vi "TestMain.vi"() -> ()   [LabVIEW 2019]
uses:
  <vilib>/Platform/TimedLoop/XDataNode/timing_clust.ctl
  <vilib>/Platform/TimedLoop/XDataNode/nitl_modes.ctl
  <vilib>/Platform/TimedLoop/XDataNode/wakeup.ctl
  <vilib>/myRIO/Instrument Drivers/Onboard IO/PWM/typedefs/PWM Reference.ctl
  <vilib>/myRIO/Common/Instrument Driver Framework/Utilities/typedefs/myRIO Generic Hardware Reference.ctl
  <vilib>/myRIO/Common/Instrument Driver Framework/Utilities/typedefs/Hardware Version Enum.ctl
  <vilib>/myRIO/Common/Instrument Driver Framework/Utilities/typedefs/myRIO v1.0 Reference.ctl
  <vilib>/myRIO/Common/Instrument Driver Framework/Utilities/typedefs/Generic FPGA Reference.ctl
  <vilib>/myRIO/Common/Instrument Driver Framework/myRIO v1.0/PWM/typedefs/PWM Channels Enum.ctl
  <vilib>/myRIO/Instrument Drivers/Onboard IO/PWM/typedefs/PWM Configuration.ctl
  <vilib>/userDefined/High Color/nirio_resource_hc.ctl
  <vilib>/myRIO/Instrument Drivers/Onboard IO/DIO/typedefs/DIO Reference.ctl
  <vilib>/myRIO/Common/Instrument Driver Framework/myRIO v1.0/DIO/typedefs/DIO Channels List.ctl
  <vilib>/myRIO/Common/Instrument Driver Framework/myRIO v1.0/DIO/typedefs/DIO Channels Enum.ctl
  <vilib>/myRIO/Common/Instrument Driver Framework/Utilities/vis/Is FPGA Ref Available.vi
  <vilib>/myRIO/Common/Instrument Driver Framework/myRIO v1.0/PWM/vis/myRIO v1.1 Open PWM.vi
  <vilib>/myRIO/Instrument Drivers/Onboard IO/PWM/vis/Set Duty Cycle and Frequency.vi
  <vilib>/myRIO/Common/Instrument Driver Framework/myRIO v1.0/DIO/vis/myRIO v1.1 Open DIO.vi
  <extravilib>/ChannelInstances/Tag-bool/Write With Abort.vi
  <extravilib>/ChannelInstances/Tag-bool/Read With Abort.vi
  <vilib>/myRIO/Common/Instrument Driver Framework/Utilities/vis/Validate Channels.vi
  <vilib>/myRIO/Common/Instrument Driver Framework/myRIO v1.0/PWM/vis/myRIO v1.0 Reserve PWM.vi
  <vilib>/myRIO/Common/Instrument Driver Framework/myRIO v1.0/DIO/vis/myRIO v1.0 Reserve DIO.vi
  <vilib>/myRIO/Common/Instrument Driver Framework/myRIO v1.0/I2C/vis/myRIO v1.0 Close I2C.vi
  <vilib>/myRIO/Common/Instrument Driver Framework/myRIO v1.0/UART/vis/myRIO v1.0 Close UART.vi
  <vilib>/myRIO/Common/Instrument Driver Framework/myRIO v1.0/PWM/vis/myRIO v1.0 Build MUX Configuration PWM.vi
  <vilib>/myRIO/Common/Instrument Driver Framework/myRIO v1.0/Resource Manager/vis/myRIO v1.0 Reserve Channel List.vi
  <vilib>/myRIO/Common/Instrument Driver Framework/myRIO v1.0/DIO/vis/myRIO v1.0 Build MUX Configuration DIO.vi
  <vilib>/myRIO/Common/Instrument Driver Framework/myRIO v1.0/I2C/vis/myRIO v1.0 Unreserve I2C.vi
  <vilib>/myRIO/Common/Instrument Driver Framework/myRIO v1.0/Resource Manager/vis/myRIO v1.0 Create Configuration List.vi
  <vilib>/myRIO/Common/Instrument Driver Framework/myRIO v1.0/Resource Manager/vis/myRIO v1.0 Reserve Channel.vi
  <vilib>/myRIO/Common/Instrument Driver Framework/myRIO v1.0/Resource Manager/vis/myRIO v1.0 Unreserve Channel.vi
  <vilib>/myRIO/Common/Instrument Driver Framework/myRIO v1.0/I2C/vis/myRIO v1.0 Build MUX Configuration I2C.vi
  <vilib>/myRIO/Common/Instrument Driver Framework/myRIO v1.0/Resource Manager/vis/myRIO v1.0 Unreserve Channel List.vi
  <vilib>/myRIO/Common/Instrument Driver Framework/myRIO v1.0/Resource Manager/vis/myRIO v1.0 Build Mutex Name.vi
  <vilib>/Instr/_visa.llb/VISA Configure Serial Port (Instr).vi
  <extravilib>/ChannelInstances/Tag-bool/Instantiate.vi
  <extravilib>/ChannelInstances/Tag-bool/EndpointRead.vi
  <vilib>/Utility/VariantDataType/GetNumericInfo.vi
  <vilib>/Utility/error.llb/Error Cluster From Error Code.vi
  <vilib>/myRIO/Common/Instrument Driver Framework/myRIO v1.0/myRIO v1.1 Open.vi
  <vilib>/myRIO/Common/Instrument Driver Framework/Utilities/vis/IO Manager.vi
  <vilib>/myRIO/Common/Instrument Driver Framework/Utilities/vis/Configuration Manager.vi
  <vilib>/myRIO/Common/Instrument Driver Framework/myRIO v1.0/Resource Manager/vis/myRIO v1.0 Configure IO.vi
  <vilib>/myRIO/Common/Instrument Driver Framework/myRIO v1.0/myRIO v1.0 Close.vi
  <vilib>/myRIO/Common/Instrument Driver Framework/myRIO v1.0/PWM/vis/myRIO v1.0 Write PWM.vi
  <vilib>/myRIO/Common/Instrument Driver Framework/myRIO v1.0/DIO/vis/myRIO v1.0 Write DIO.vi
  <vilib>/myRIO/Common/Instrument Driver Framework/myRIO v1.0/I2C/vis/myRIO v1.0 Shutdown I2C.vi
  <vilib>/rvi/errors/niLvFpgaAdjustHostInterfaceError.vi
  <vilib>/FPGAPlugInAG/Dynamic/niLvFpga_Abort_Dynamic.vi
  <vilib>/myRIO/Common/Instrument Driver Framework/Utilities/vis/FPGA Ref Manager.vi
  <vilib>/myRIO/Common/Instrument Driver Framework/myRIO v1.0/myRIO v1.0 Reset FPGA.vi
  <vilib>/myRIO/Common/Instrument Driver Framework/myRIO v1.0/IRQ/vis/myRIO v1.0 IRQ Info FGV.vi
  <vilib>/myRIO/Common/Instrument Driver Framework/myRIO v1.0/IRQ/vis/myRIO v1.0 Timer IRQ Info FGV.vi
  <vilib>/myRIO/Common/Instrument Driver Framework/myRIO v1.0/IRQ/vis/myRIO v1.0 ISR Agent.vi
  <vilib>/myRIO/Instrument Drivers/Utilities/vis/Reset Index.vi
  <vilib>/myRIO/Common/Instrument Driver Framework/myRIO v1.0/Resource Manager/vis/myRIO v1.0 Block Write Resource Manager.vi
  <vilib>/FPGAPlugInAG/Dynamic/niLvFpga_Close_Dynamic.vi
  <extravilib>/ChannelInstances/Tag-bool/Endpoint.vi
  <vilib>/platform/TimedLoop/XDataNode/XDataNode.xnode
  <vilib>/myRIO/Express VI/Onboard IO/PWM/PWM Express VI.xnode
  <vilib>/myRIO/Instrument Drivers/Onboard IO/PWM/vis/myRIO PWM Open.xnode
  <vilib>/myRIO/Express VI/Onboard IO/DO/DO Express VI.xnode
  <vilib>/myRIO/Instrument Drivers/Onboard IO/DIO/vis/myRIO DIO Open.xnode
  <vilib>/rvi/interface/nirviReadWriteControl/nirviReadWriteControl.xnode
  <vilib>/rvi/interface/nirviMethod/nirviMethod.xnode
  <vilib>/rvi/interface/nirviCloseFPGA/nirviCloseFPGA.xnode
  <vilib>/rvi/interface/Simulation/niFpgaSimulationCallBeginRW.vi
  <vilib>/Platform/TimedLoop/XDataNode/XDNodeRunTimeDep.lvlib
  <vilib>/myRIO/Instrument Drivers/Utilities/Utilities.lvlib
  NiFpgaLv.dll
  <extravilib>/ChannelInstances/Tag-bool.lvlib
  <vilib>/myRIO/Instrument Drivers/Onboard IO/PWM/PWM.lvlib
  <vilib>/myRIO/Instrument Drivers/Onboard IO/DIO/DIO.lvlib
  <vilib>/myRIO/Instrument Drivers/Onboard IO/I2C/I2C.lvlib
panel:
  in  "Log file path":path
  out "Duty Cycle":dbl
  in  "Angle limit":i32
  in  "D":dbl
  in  "I":dbl
  in  "P":dbl
  in  "Speed (rpm)":i32
  out "Raw output from GPS":string
  in  "Organised Output from the GPS":T1(tab)
  out "GPGSV":string
  out "number of message":string
  out "msg1":string
  out "Satelite in view":string
  in  "Satelite_id/elevation/azimuth/SNR 17":enum32{"Msg 1", "Msg 2", "Msg 3", "Msg 4"}(tab)
  out "Satelite_id/elevation/azimuth/SNR":string[](array[string])
  out "Satelite_id/elevation/azimuth/SNR 2":string[](array[string])
  out "Satelite_id/elevation/azimuth/SNR 3":string[](array[string])
  out "Satelite_id/elevation/azimuth/SNR 4":string[](array[string])
  out "Signal ID / Check sum":string[](array[string])
  out "Signal ID / Check sum 2":string[](array[string])
  out "Satelite_id/elevation/azimuth/SNR 8":string[](array[string])
  out "Satelite_id/elevation/azimuth/SNR 7":string[](array[string])
  out "Satelite_id/elevation/azimuth/SNR 6":string[](array[string])
  out "Satelite_id/elevation/azimuth/SNR 5":string[](array[string])
  out "Signal ID / Check sum 3":string[](array[string])
  out "Satelite_id/elevation/azimuth/SNR 12":string[](array[string])
  out "Satelite_id/elevation/azimuth/SNR 11":string[](array[string])
  out "Satelite_id/elevation/azimuth/SNR 10":string[](array[string])
  out "Satelite_id/elevation/azimuth/SNR 9":string[](array[string])
  out "Signal ID / Check sum 4":string[](array[string])
  out "Satelite_id/elevation/azimuth/SNR 16":string[](array[string])
  out "Satelite_id/elevation/azimuth/SNR 15":string[](array[string])
  out "Satelite_id/elevation/azimuth/SNR 14":string[](array[string])
  out "Satelite_id/elevation/azimuth/SNR 13":string[](array[string])
  out "GLGSV 2":string
  out "number of message 2":string
  out "msg1 2":string
  out "Satelite in view 2":string
  in  "Satelite_id/elevation/azimuth/SNR 34":enum32{"Msg 1", "Msg 2", "Msg 3", "Msg 4"}(tab)
  out "Satelite_id/elevation/azimuth/SNR 21":string[](array[string])
  out "Satelite_id/elevation/azimuth/SNR 20":string[](array[string])
  out "Satelite_id/elevation/azimuth/SNR 19":string[](array[string])
  out "Satelite_id/elevation/azimuth/SNR 18":string[](array[string])
  out "Signal ID / Check sum 5":string[](array[string])
  out "Signal ID / Check sum 6":string[](array[string])
  out "Satelite_id/elevation/azimuth/SNR 25":string[](array[string])
  out "Satelite_id/elevation/azimuth/SNR 22":string[](array[string])
  out "Satelite_id/elevation/azimuth/SNR 23":string[](array[string])
  out "Satelite_id/elevation/azimuth/SNR 24":string[](array[string])
  out "Signal ID / Check sum 7":string[](array[string])
  out "Satelite_id/elevation/azimuth/SNR 29":string[](array[string])
  out "Satelite_id/elevation/azimuth/SNR 26":string[](array[string])
  out "Satelite_id/elevation/azimuth/SNR 27":string[](array[string])
  out "Satelite_id/elevation/azimuth/SNR 28":string[](array[string])
  out "Signal ID / Check sum 8":string[](array[string])
  out "Satelite_id/elevation/azimuth/SNR 33":string[](array[string])
  out "Satelite_id/elevation/azimuth/SNR 30":string[](array[string])
  out "Satelite_id/elevation/azimuth/SNR 31":string[](array[string])
  out "Satelite_id/elevation/azimuth/SNR 32":string[](array[string])
  out "GAGSV 3":string
  out "number of message 3":string
  out "msg1 3":string
  out "Satelite in view 3":string
  in  "Satelite_id/elevation/azimuth/SNR 51":enum32{"Msg 1", "Msg 2", "Msg 3", "Msg 4"}(tab)
  out "Satelite_id/elevation/azimuth/SNR 38":string[](array[string])
  out "Satelite_id/elevation/azimuth/SNR 37":string[](array[string])
  out "Satelite_id/elevation/azimuth/SNR 36":string[](array[string])
  out "Satelite_id/elevation/azimuth/SNR 35":string[](array[string])
  out "Signal ID / Check sum 9":string[](array[string])
  out "Signal ID / Check sum 10":string[](array[string])
  out "Satelite_id/elevation/azimuth/SNR 42":string[](array[string])
  out "Satelite_id/elevation/azimuth/SNR 39":string[](array[string])
  out "Satelite_id/elevation/azimuth/SNR 40":string[](array[string])
  out "Satelite_id/elevation/azimuth/SNR 41":string[](array[string])
  out "Signal ID / Check sum 11":string[](array[string])
  out "Satelite_id/elevation/azimuth/SNR 46":string[](array[string])
  out "Satelite_id/elevation/azimuth/SNR 43":string[](array[string])
  out "Satelite_id/elevation/azimuth/SNR 44":string[](array[string])
  out "Satelite_id/elevation/azimuth/SNR 45":string[](array[string])
  out "Signal ID / Check sum 12":string[](array[string])
  out "Satelite_id/elevation/azimuth/SNR 50":string[](array[string])
  out "Satelite_id/elevation/azimuth/SNR 47":string[](array[string])
  out "Satelite_id/elevation/azimuth/SNR 48":string[](array[string])
  out "Satelite_id/elevation/azimuth/SNR 49":string[](array[string])
  out "GBGSV 4":string
  out "number of message 4":string
  out "msg1 4":string
  out "Satelite in view 4":string
  in  "Satelite_id/elevation/azimuth/SNR 68":enum32{"Msg 1", "Msg 2", "Msg 3", "Msg 4"}(tab)
  out "Satelite_id/elevation/azimuth/SNR 55":string[](array[string])
  out "Satelite_id/elevation/azimuth/SNR 54":string[](array[string])
  out "Satelite_id/elevation/azimuth/SNR 53":string[](array[string])
  out "Satelite_id/elevation/azimuth/SNR 52":string[](array[string])
  out "Signal ID / Check sum 13":string[](array[string])
  out "Signal ID / Check sum 14":string[](array[string])
  out "Satelite_id/elevation/azimuth/SNR 59":string[](array[string])
  out "Satelite_id/elevation/azimuth/SNR 56":string[](array[string])
  out "Satelite_id/elevation/azimuth/SNR 57":string[](array[string])
  out "Satelite_id/elevation/azimuth/SNR 58":string[](array[string])
  out "Signal ID / Check sum 15":string[](array[string])
  out "Satelite_id/elevation/azimuth/SNR 63":string[](array[string])
  out "Satelite_id/elevation/azimuth/SNR 60":string[](array[string])
  out "Satelite_id/elevation/azimuth/SNR 61":string[](array[string])
  out "Satelite_id/elevation/azimuth/SNR 62":string[](array[string])
  out "Signal ID / Check sum 16":string[](array[string])
  out "Satelite_id/elevation/azimuth/SNR 67":string[](array[string])
  out "Satelite_id/elevation/azimuth/SNR 64":string[](array[string])
  out "Satelite_id/elevation/azimuth/SNR 65":string[](array[string])
  out "Satelite_id/elevation/azimuth/SNR 66":string[](array[string])
  out "UTC Time":string
  out "N/S":string
  out "Long":string
  out "Mode":string
  out "Status":string
  out "Lat":string
  out "Course over Ground [Degrees]":string
  out "date[ddmmyy]":string
  out "E/W":string
  out "Speed over ground[knot]":string
  out "xxRMC":string
  out "NavStatus":string
  out "Checksum":string
  out "Carriage return":string
  out "Lat 2":string
  out "NS":string
  out "GLL":string
  out "Long 3":string
  out "EW":string
  out "Time":string
  out "Status 2":string
  out "Positioning mod":string
  out "Check sum":string
  out "Carriage return 2":string
  out "VTG":string
  out "Course over Ground":string
  out "Reference":string
  out "Course over Ground (Magnetic)":string
  out "Reference2":string
  out "Speedover Ground (knots)":string
  out "Units1":string
  out "Speed over ground kph":string
  out "Units 2":string
  out "Position Mode 2":string
  out "Check sum 2":string
  out "GGA 3":string
  out "UTC time":string
  out "Lat 3":string
  out "NS 2":string
  out "Long 2":string
  out "EW 2":string
  out "Pos_indicator":string
  out "Number of Satelite_used":string
  out "hdop":string
  out "msl_altitude":string
  out "altitude_units":string
  out "geoidal_Seperation":string
  out "Separation unit":string
  out "age of Diff corr":string
  out "diffStating":string
  out "Checksum 2":string
  out "GSA":string
  out "Operation Mode":string
  out "Navigation mode":string
  out "satelite used channel 1":string
  out "satelite used channel 3":string
  out "satelite used channel 4":string
  out "satelite used channel 5":string
  out "satelite used channel 6":string
  out "satelite used channel 7":string
  out "satelite used channel 8":string
  out "satelite used channel 9":string
  out "satelite used channel 10":string
  out "satelite used channel 11":string
  out "satelite used channel 12":string
  out "pdop":string
  out "hdop 2":string
  out "vdop":string
  out "System ID":string
  out "Checksum 3":string
  out "satelite used channel 2":string
  out "Combined loop duration time (us)":i64
  in  "Loop durations":T2(tab)
  out "IMU Data gathering duration(us)":i64(graph)
  out "Hall data gathering duration(us)":i64(graph)
  out "Encoder data gathering duration(us)":i64(graph)
  out "Steering Motor duration(us)":i64(graph)
  out "E-Stop loop duration (us)":i64(graph)
  out "GPS loop duration (us)":i64(graph)
  in  "GO":bool
  in  "E-stop":bool
  out "Indicator":bool
  in  "Encoder Position Reset":bool
  out "Encoder Velocity (Counts/Interval)":i32
  out "Encoder Acceleration (Counts/Interval)":i32
  out "Encoder Position (Counts)":i32
  out "Hall Detection":bool
  out "Hall Period":u32
  out "IMU Gyro Chart":cluster{dbl, dbl, dbl}(graph)
  out "IMU Acc Chart":cluster{dbl, dbl, dbl}(graph)
  # "Steering Motor"
  # "Forward Motor"
  # "Start Motors"
  # "Signal ID / Check sum"
  # "Signal ID / Check sum"
  # "Signal ID / Check sum"
  # "Signal ID / Check sum"
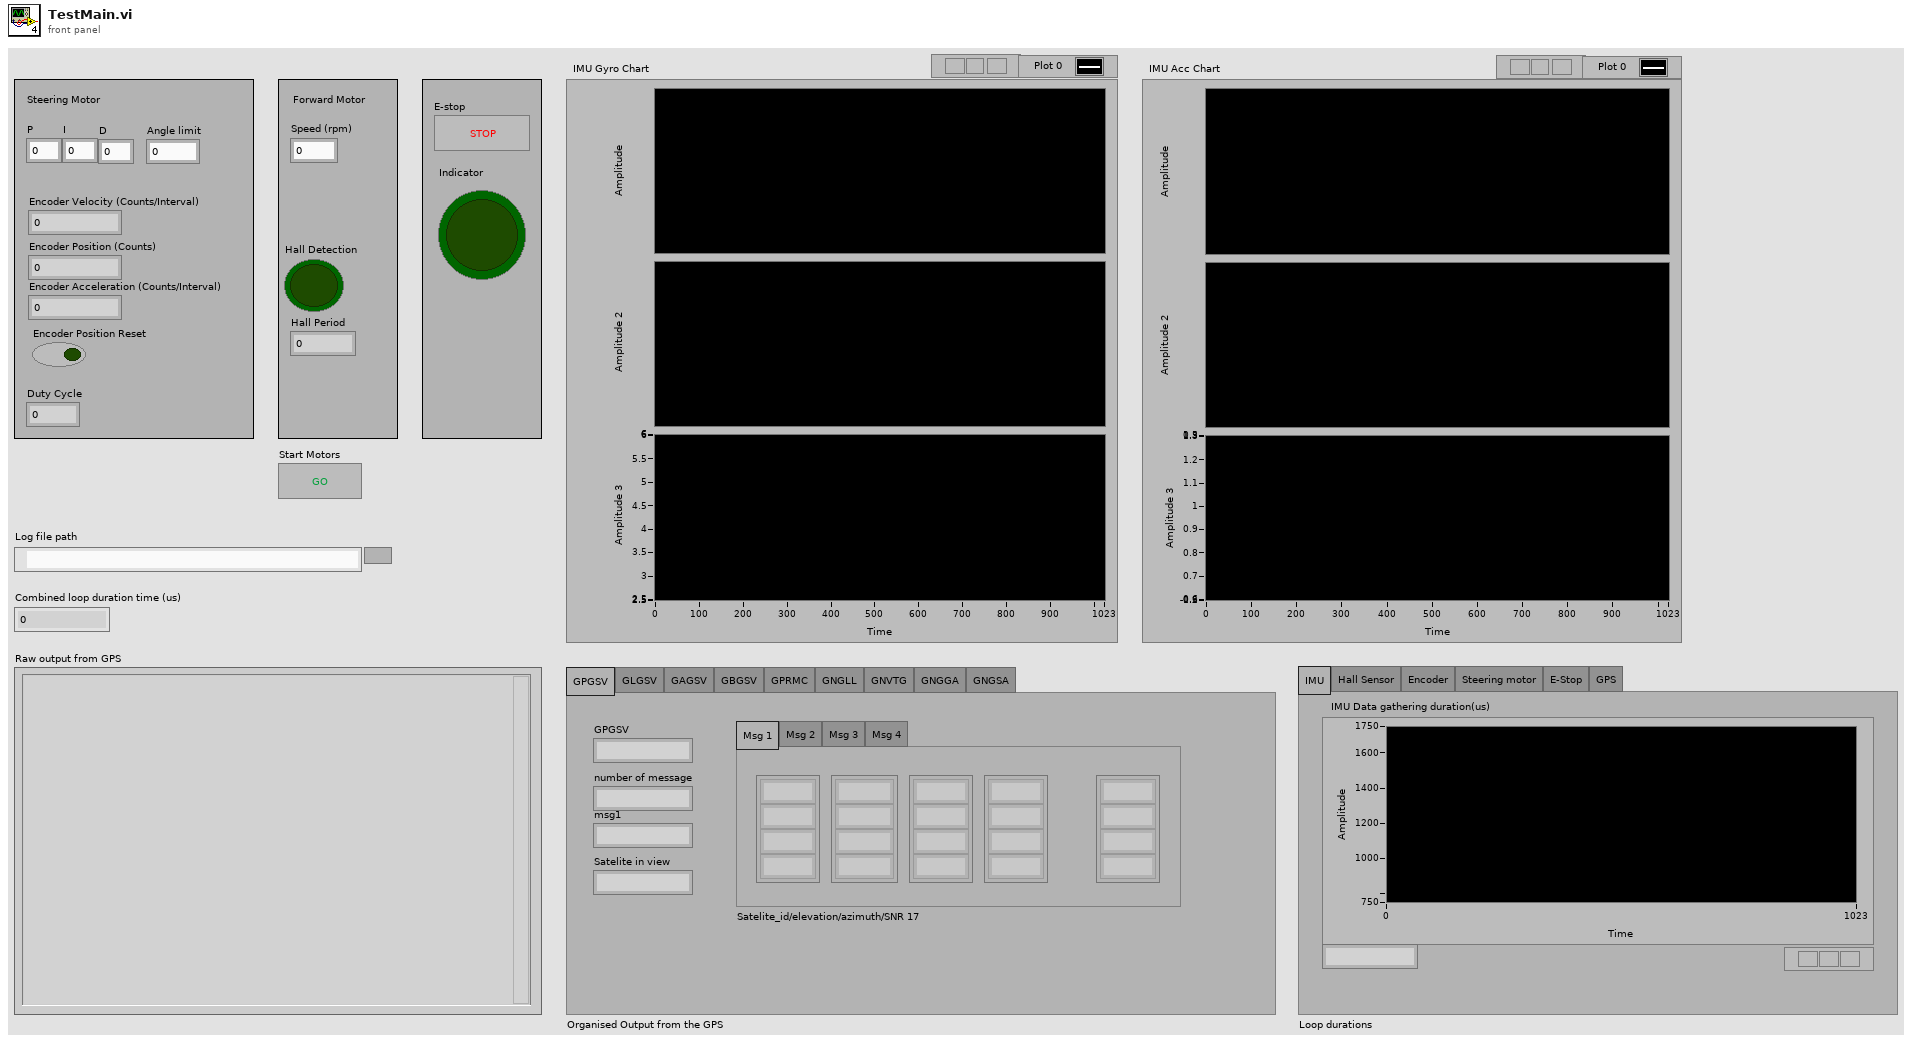
[diagram p1: front panel]
types:
  T1 = enum32{"GPGSV", "GLGSV", "GAGSV", "GBGSV", "GPRMC", "GNGLL", "GNVTG", "GNGGA", "GNGSA"}
  T2 = enum32{"IMU", "Hall Sensor", "Encoder", "Steering motor", "E-Stop", "GPS"}
  T3 = enum16{"open", "open or create", "create or replace", "create", "open (read-only)"}
  T4 = typedef "I2C.lvlib/I2C Reference.ctl" = cluster{"myRIO Reference":T5, "I2C Channels Enum":T9, "I2C Configuration":T10}
  T5 = typedef "myRIO Generic Hardware Reference.ctl" = cluster{"myRIO Model":T6, "myRIO Hardware Reference":T7}
  T6 = typedef "Hardware Version Enum.ctl" = enum16{"Unknown", "myRIO-1900", "myRIO-1950", "roboRIO", "NI ELVIS RIO CM", "ELVIS III"}
  T7 = typedef "myRIO v1.0 Reference.ctl" = cluster{"Generic FPGA Reference":T8, "Allow multiple opens":bool}
  T8 = typedef "Generic FPGA Reference.ctl" = refnum<k20>
  T9 = typedef "I2C Channels Enum.ctl" = enum16{"Not Connected", "A/I2C", "B/I2C", "I2C/I2C"}
  T10 = typedef "I2C.lvlib/I2C Configuration.ctl" = cluster{"I2C Transfer Rate":T11}
  T11 = typedef "I2C.lvlib/I2C Transfer Rate.ctl" = enum16{"Standard mode (100 kbps)", "Fast mode (400 kbps)"}
  T12 = typedef "XDNodeRunTimeDep.lvlib/timing_clust.ctl" = cluster{"Expected End [f-1]":u64, "Actual End [f-1]":u64, "Finished Late? [f-1]":bool, "Expected End [i-1]":u64, "Actual End [i-1]":u64, "Finished Late? [i-1]":bool, "Expected Start [i]":u64, "Actual Start [i]":u64, "Expected Start [f]":u64, "Actual Start [f]":u64, "Source Name":string, "Structure Name":string, "Period":i64, "Deadline":i64, "Offset":i64, "Start":i64, "Priority":i32, "Timeout":i32, "Mode":T13, "Wakeup Reason":T14, "Error":errorcluster, "Source Type":string, "Secondary Source Type":string, "Global End Time":u64, "Global Start Time":u64, "Frame Duration":u64, "Iteration Duration":u64, "Assigned CPU":i32, "I/O Scan Engine Mode":u32}
  T13 = typedef "XDNodeRunTimeDep.lvlib/nitl_modes.ctl" = enum32{"No Change", "Process missed periods, maintain original phase", "Discard missed periods, maintain original phase", "Process missed periods, ignore original phase", "Discard missed periods, ignore original phase"}
  T14 = typedef "XDNodeRunTimeDep.lvlib/wakeup.ctl" = enum32{"Normal", "Aborted", "Asynchronous wakeup", "Timing source error", "Timed loop error", "Timeout"}
  T15 = typedef "Tag-bool.lvlib/))Channel.ctl" = refnum<queue>
  T16 = typedef "PWM.lvlib/PWM Reference.ctl" = cluster{"myRIO Reference":T5, "PWM Channels Enum":T17, "PWM Configuration":T18}
  T17 = typedef "PWM Channels Enum.ctl" = enum16{"Not Connected", "C/PWM0", "C/PWM1", "A/PWM0", "A/PWM1", "A/PWM2", "A/PWM3", "A/PWM4", "A/PWM5", "A/PWM6", "A/PWM7", "A/PWM8", "A/PWM9", "A/PWM10", "A/PWM11", "A/PWM12", "A/PWM13", "A/PWM14", "A/PWM15", "A/PWM16", "A/PWM17", "A/PWM18", "A/PWM19", "B/PWM0", "B/PWM1", "B/PWM2", "B/PWM3", "B/PWM4", "B/PWM5", "B/PWM6", "B/PWM7", "B/PWM8", "B/PWM9", "B/PWM10", "B/PWM11", "B/PWM12", "B/PWM13", "B/PWM14", "B/PWM15", "B/PWM16", "B/PWM17", "B/PWM18", "B/PWM19", "PWM/PWM0", "PWM/PWM1", "PWM/PWM2", "PWM/PWM3", "PWM/PWM4", "PWM/PWM5", "PWM/PWM6", "PWM/PWM7", "PWM/PWM8", "PWM/PWM9"}
  T18 = typedef "PWM.lvlib/PWM Configuration.ctl" = cluster{"Frequency":dbl, "Duty Cycle":dbl}
  T19 = typedef "nirio_resource_hc.ctl" = tag
  T20 = typedef "DIO.lvlib/DIO Reference.ctl" = cluster{"myRIO Reference":T5, "DIO Channels List":T21}
  T21 = typedef "DIO Channels List.ctl" = T22[]
  T22 = typedef "DIO Channels Enum.ctl" = enum16{"Not Connected", "C/DIO0", "C/DIO1", "C/DIO2", "C/DIO3", "C/DIO4", "C/DIO5", "C/DIO6", "C/DIO7", "A/DIO0", "A/DIO1", "A/DIO2", "A/DIO3", "A/DIO4", "A/DIO5", "A/DIO6", "A/DIO7", "A/DIO8", "A/DIO9", "A/DIO10", "A/DIO11", "A/DIO12", "A/DIO13", "A/DIO14", "A/DIO15", "A/DIO16", "A/DIO17", "A/DIO18", "A/DIO19", "B/DIO0", "B/DIO1", "B/DIO2", "B/DIO3", "B/DIO4", "B/DIO5", "B/DIO6", "B/DIO7", "B/DIO8", "B/DIO9", "B/DIO10", "B/DIO11", "B/DIO12", "B/DIO13", "B/DIO14", "B/DIO15", "B/DIO16", "B/DIO17", "B/DIO18", "B/DIO19", "LED0", "LED1", "LED2", "LED3", "Button0", "DIO/DIO0", "DIO/DIO1", "DIO/DIO2", "DIO/DIO3", "DIO/DIO4", "DIO/DIO5", "DIO/DIO6", "DIO/DIO7", "DIO/DIO8", "DIO/DIO9", "SPI/CS0", "SPI/CS1", "SPI/CS2", "SPI/CS3", "LED RADIO (Green)", "LED RADIO (Red)", "LED COMM (Green)", "LED COMM (Red)", "LED MODE (Green)", "LED MODE (Red)"}
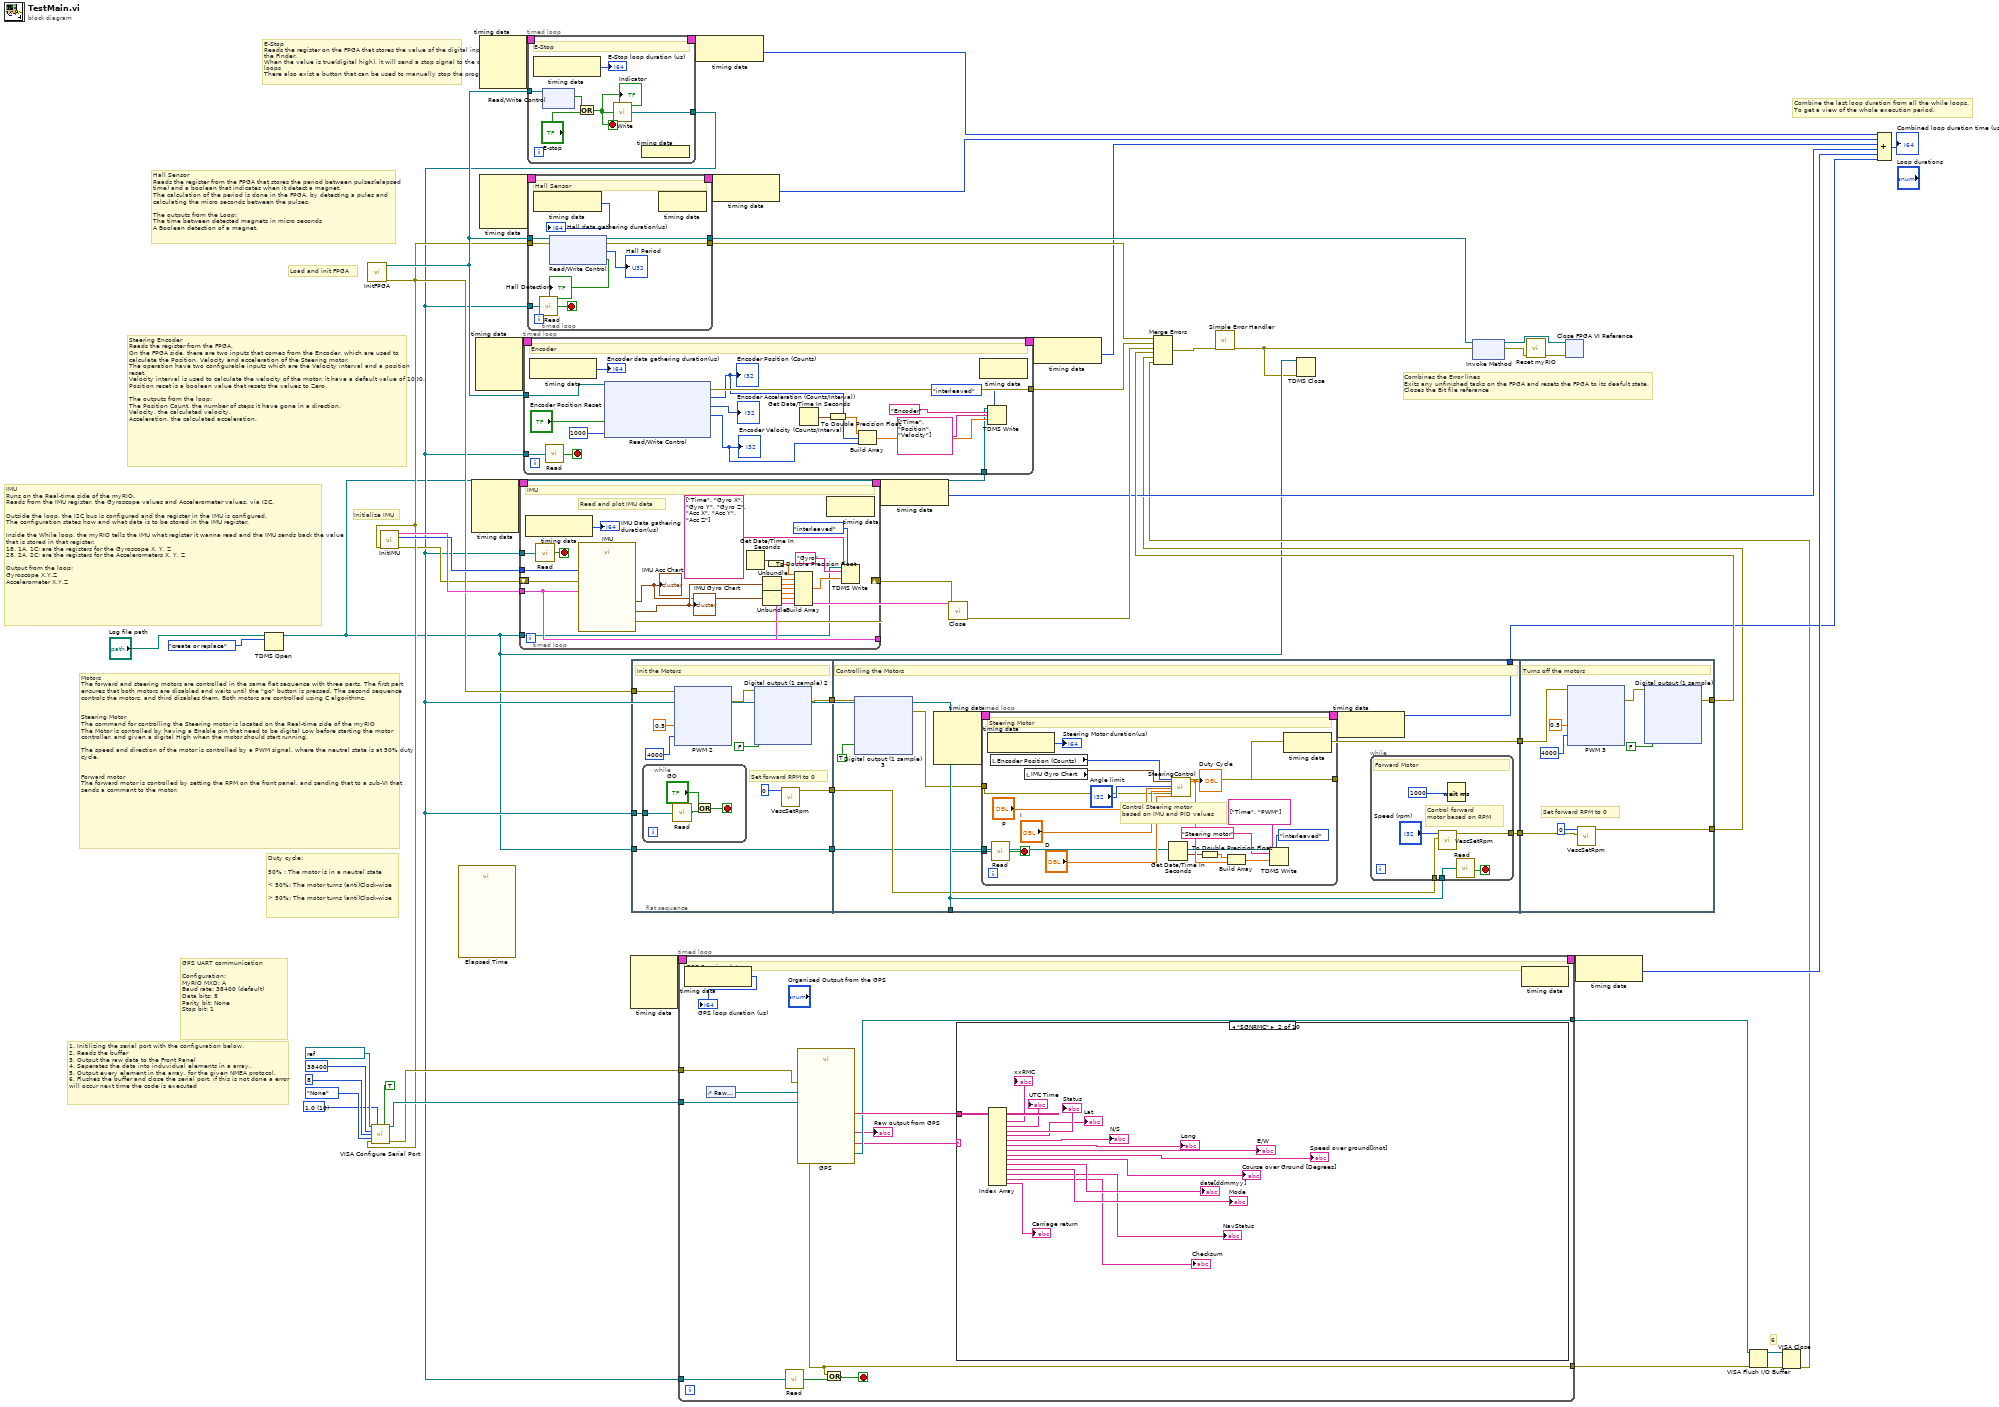
[diagram p0: block diagram]
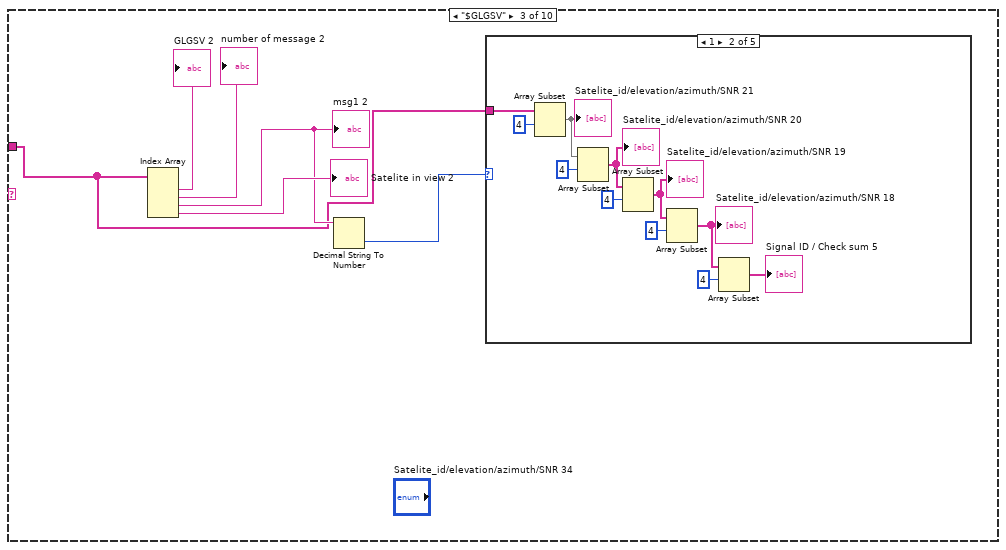
[diagram p3: hidden frame]
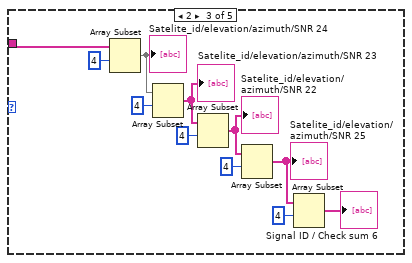
[diagram p5: hidden frame]
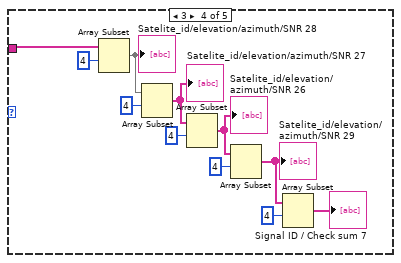
[diagram p6: hidden frame]
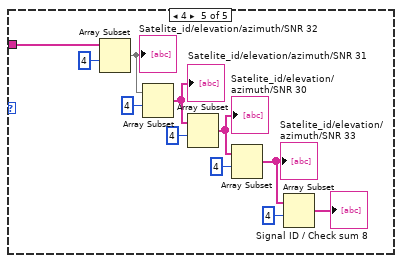
[diagram p7: hidden frame]
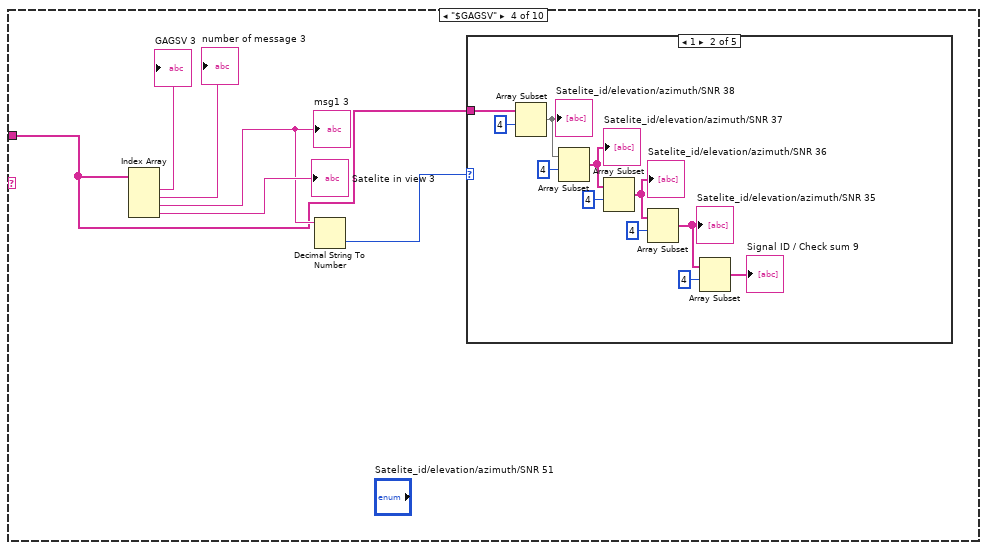
[diagram p8: hidden frame]
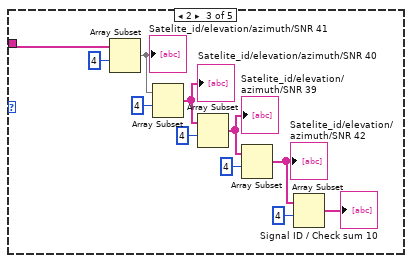
[diagram p10: hidden frame]
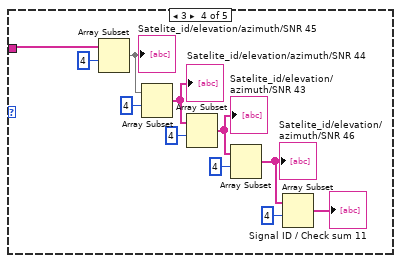
[diagram p11: hidden frame]
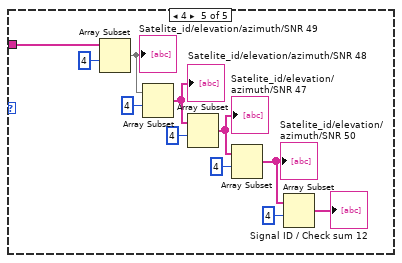
[diagram p12: hidden frame]
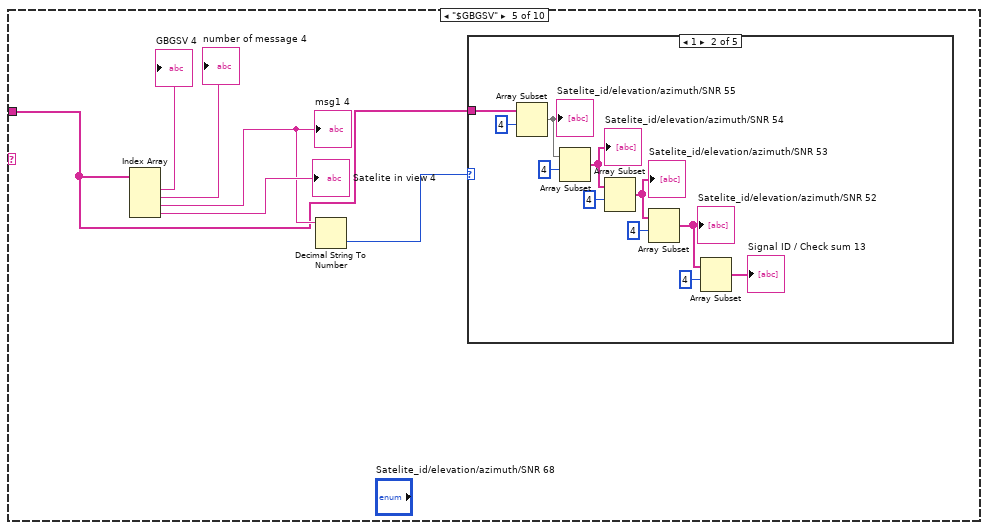
[diagram p13: hidden frame]
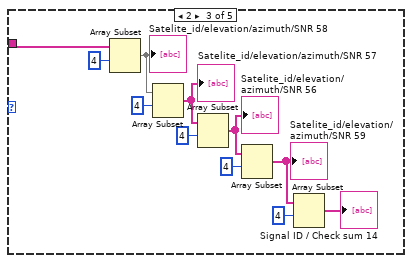
[diagram p15: hidden frame]
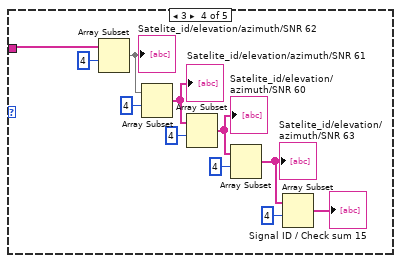
[diagram p16: hidden frame]
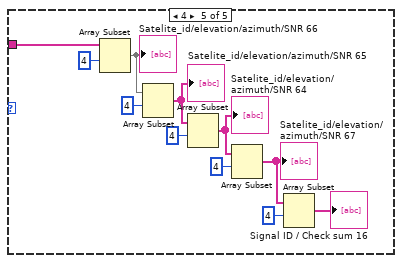
[diagram p17: hidden frame]
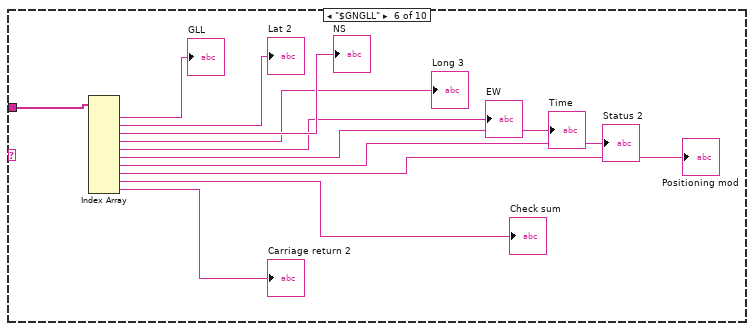
[diagram p18: hidden frame]
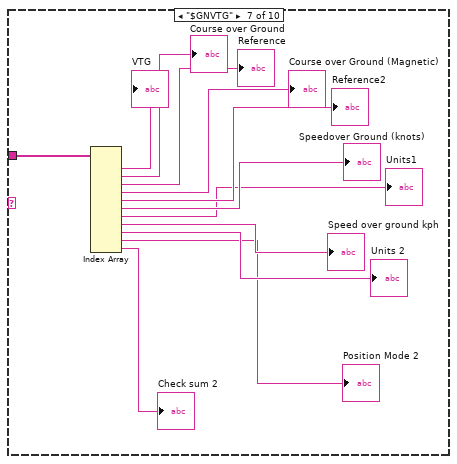
[diagram p19: hidden frame]
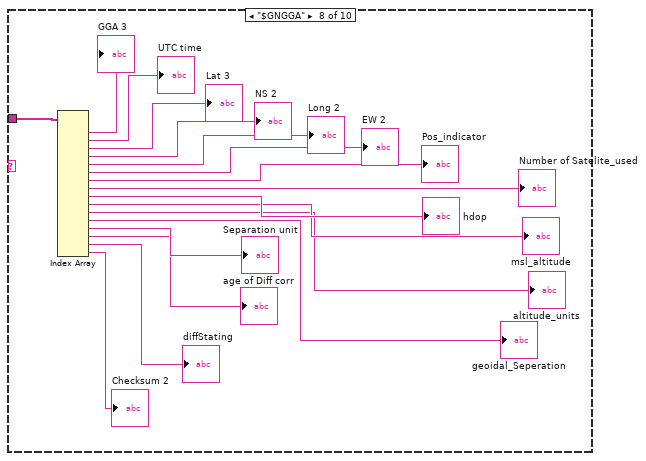
[diagram p20: hidden frame]
diagram:
  w27 = u16 10 items=["1.0"=10, "1.5"=15, "2.0"=20] ("stop bits (10: 1 bit)")
  # "Duty cycle:\n\n50% : The motor is in a neutral state\n\n< 50%: The motor turns (anti)Clock-wise\n\n> 50%: The motor turns (anti)Clock-wise"
  # "Initialize IMU"
  # "Load and init FPGA"
  # "Combines the Error lines\nExits any unfinished tasks on the FPGA and resets the FPGA to its deafult state.\nCloses the Bit file referance"
  # "Combine the last loop duration from all the while loops.\nTo get a view of the whole execution period."
  # "1. Initilizing the serial port with the configuration below.\n2. Reads the buffer\n3. Output the raw data to the Front Panel\n4. Seperates the data into induvidual elements in a array.\n5. Output every element in the array, for the given NMEA protocol.\n6. Flushes the buffer and close the serial port, if this is not done a error will occur next time the code is executed"
  # "Motors\nThe forward and steering motors are controlled in the same flat sequence with three parts. The first part ensures that both motors are disabled and waits until the \"go\" button is pressed. The second sequence controls the motors, and third disables them. Both motors are controlled using C algorithms.\n\n\nSteering Motor\nThe command for controlling the Steering motor is located on the Real-time side of the myRIO\nThe Motor is controlled by having a Enable pin that need to be digital Low before starting the motor controller, and given a digital High when the motor should start running.\n\nThe speed and direction of the motor is controlled by a PWM signal, where the neutral state is at 50% duty cycle.\n\n\nForward motor\nThe forward motor is controlled by setting the RPM on the front panel, and sending that to a sub-VI that sends a commant to the motor."
  # "IMU\nRuns on the Real-time side of the myRIO.\nReads from the IMU register, the Gyroscope values and Accelerometer values, via I2C.\n\nOutside the loop, the I2C bus is configured and the register in the IMU is configured.\nThe configuration states how and what data is to be stored in the IMU register.\n\nInside the While loop, the myRIO tells the IMU what register it wanna read and the IMU sends back the value that is stored in that register.\n18, 1A, 1C: are the registers for the Gyroscope X, Y, Z\n28, 2A, 2C: are the registers for the Accelerometers X, Y, Z\n\nOutput from the loop:\nGyroscope X,Y,Z\nAccelerometer X,Y,Z"
  # "Steering Encoder\nReads the register from the FPGA. \nOn the FPGA side, there are two inputs that comes from the Encoder, which are used to calculate the Position, Velocity and acceleration of the Steering motor.\nThe operation have two configurable inputs which are the Velocity interval and a position reset.\nVelocity interval is used to calculate the velocity of the motor, it have a default value of 1000.\nPosition reset is a boolean value that resets the values to Zero.\n\nThe outputs from the loop:\nThe Position Count, the number of steps it have gone in a direction. \nVelocity, the calculated velocity.\nAcceleration, the calculated acceleration."
  # "Hall Sensor\nReads the register from the FPGA that stores the period between pulses(elapsed time) and a boolean that indicates when it detect a magnet.\nThe calculation of the period is done in the FPGA, by detecting a pules and calculating the micro seconds between the pulses.\n\nThe outputs from the Loop:\nThe time between detected magnets in micro seconds\nA Boolean detection of a magnet."
  # "E-Stop\nReads the register on the FPGA that stores the value of the digital input from the Finder.\nWhen the value is true(digital high), it will send a stop signal to the other while loops\nThere also exist a button that can be used to manually stop the program."
  # "6"
  # "GPS UART communication\n\nConfiguration:\nMyRIO MXD: A\nBaud rate: 38400 (default)\nData bits: 8\nParity bit: None\nStop bit: 1"
  n1 = TDMS Open(10:T3."create or replace" ("operation (0:open)"), 11:"Log file path") -> (3:w2:refnum<k34>)  [unwired: 5 in, 1 out]
  n2 = call "InitFPGA.vi"() -> ("error out"=w21:errorcluster, "Refnum out"=w35:refnum<k20>)  [unwired: 10 in]
  n3 = call-poly "VISA Configure Serial Port"("VISA resource name"=refnum<visa-resource-name> "ASRL1::INSTR", "Enable Termination\nChar (T)"=TRUE ("Enable Termination\nChar (T)"), "baud rate (9600)"=u32 38400, "data bits (8)"=u16 8, "parity (0:none)"=enum16{"None", "Odd", "Even", "Mark", "Space"}."None", "error in (no error)"=w21, "stop bits (10: 1 bit)"=w27) -> ("VISA resource name out"=w24:refnum<visa-resource-name>, "error out"=w23:errorcluster)  [unwired: 7 in]
  n4 = call "InitIMU.vi"("error in (no error)"=w21) -> ("error out"=w15:errorcluster, "Acc/Gyro  address"=w37:u8, "I2C Ref Out"=w36:T4)  [unwired: 8 in]
  n5 = call "Elapsed Time"() -> ()  [unwired: 12 in, 8 out]
  n6 = node-c288() -> (w46:T12)  [unwired: 4 in]
  n7 = node-c288() -> (w51:T12)  [unwired: 4 in]
  n8 = node-c288() -> (w44:T12)  [unwired: 4 in]
  n9 = node-c288() -> (w53:T12)  [unwired: 4 in]
  n10 = timed-loop {
    timing: w44 -> [_]
    timing-out: [_] -> w43
    tunnel: w35 -> [w63]
    tunnel: [w62] -> w11
    stop <- w58 stop-if-true
    # "E-Stop"
    n11 = node-c288() -> (→"E-Stop loop duration (us)":i64)  [unwired: 1 in]
    n12 = xnode "Read/Write Control"("FPGA VI Reference In"=w63) -> ("E-Stop"=w61:bool)  [unwired: 1 in, 2 out]
    n13 = Or(x=w61, y="E-stop") -> (x .or. y?=w58:bool)
    "Indicator" <- w58
    n14 = call <vilib>:"Write.vi"("element"=w58) -> ("channel"=w62:T15)  [unwired: 1 out]
    n15 = node-c288() -> ()  [unwired: 1 out]
  }
  n16 = timed-loop {
    timing: w46 -> [_]
    timing-out: [_] -> w45
    tunnel: w37 -> [w88]
    tunnel: w36 -> [w85]
    shift-right: [w82] -> w16
    shift-left: w15 -> [w87]
    tunnel: [w85] -> w20
    tunnel: w11 -> [w84]
    tunnel: w2 -> [w77]
    stop <- w83 stop-if-true
    # "Read and plot IMU data"
    # "IMU"
    n17 = node-c288() -> (→"IMU Data gathering duration(us)":i64)  [unwired: 1 in]
    n18 = call <extravilib>:"Read.vi"("channel"=w84) -> ("element"=w83:bool)  [unwired: 1 in, 1 out]
    n19 = call "IMU.vi"("error in (no error)"=w87, "Acc/Gyro  address"=w88, "I2C Ref"=w85) -> ("error out"=w82:errorcluster, "IMU Acc"=w70:cluster{dbl, dbl, dbl}, "IMU Gyro"=w81:cluster{dbl, dbl, dbl})  [unwired: 6 in]
    "IMU Acc Chart" <- w70
    "IMU Gyro Chart" <- w81
    n20 = Get Date/Time In Seconds() -> (seconds since 1Jan1904=w75:timestamp)
    n21 = Unbundle(w81) -> (w80:dbl, w72:dbl, w71:dbl)
    n22 = Unbundle(w70) -> (w69:dbl, w68:dbl, w67:dbl)
    n23 = To Double Precision Float(number=w75) -> (double precision float=w76:dbl)
    n24 = Build Array(w76, w80, w72, w71, w69, w68, w67) -> (w78:dbl[])
    n25 = node-c288() -> ()  [unwired: 1 in, 1 out]
    n26 = TDMS Write(0:w77, 1:enum16{"decimated", "interleaved"}."interleaved" ("data layout (0:decimated)"), 5:"Gyro" ("group name in (Untitled)"), 7:string[] ["Time", "Gyro X", "Gyro Y", "Gyro Z", "Acc X", "Acc Y", "Acc Z"] ("channel name(s) in (Untitled)"), 9:w78) -> ()  [unwired: 1 in, 4 out]
  }
  n27 = timed-loop {
    timing: w51 -> [_]
    timing-out: [_] -> w50
    tunnel: w35 -> [w108]
    tunnel: [w107] -> w48
    tunnel: w11 -> [w102]
    tunnel: w2 -> [w95]
    stop <- w101 stop-if-true
    # "Encoder"
    n28 = node-c288() -> (→"Encoder data gathering duration(us)":i64)  [unwired: 1 in]
    n29 = call <extravilib>:"Read.vi"("channel"=w102) -> ("element"=w101:bool)  [unwired: 1 in, 1 out]
    n30 = xnode "Read/Write Control"("FPGA VI Reference In"=w108, "Position Reset"="Encoder Position Reset", "Velocity Interval (uSec)"=u32 1000) -> ("error out"=w107:errorcluster, "Position (Counts)"=w98:i32, "Acceleration (Counts/Interval)"=→"Encoder Acceleration (Counts/Interval)":i32, "Velocity (Counts/Interval)"=w97:i32)  [unwired: 1 in, 1 out]
    "Encoder Position (Counts)" <- w98
    "Encoder Velocity (Counts/Interval)" <- w97
    n31 = Get Date/Time In Seconds() -> (seconds since 1Jan1904=w93:timestamp)
    n32 = To Double Precision Float(number=w93) -> (double precision float=w94:dbl)
    n33 = Build Array(w94, w98, w97) -> (w96:dbl[])
    n34 = node-c288() -> ()  [unwired: 1 in, 1 out]
    n35 = TDMS Write(0:w95, 1:enum16{"decimated", "interleaved"}."interleaved" ("data layout (0:decimated)"), 5:"Encoder" ("group name in (Untitled)"), 7:string[] ["Time", "Position", "Velocity"] ("channel name(s) in (Untitled)"), 9:w96) -> ()  [unwired: 1 in, 4 out]
  }
  n36 = timed-loop {
    tunnel: w21 -> [w120]
    tunnel: w35 -> [w119]
    tunnel: [w117] -> w54
    tunnel: [w116] -> w49
    timing: w53 -> [_]
    timing-out: [_] -> w52
    tunnel: w11 -> [w113]
    stop <- w112 stop-if-true
    # "Hall Sensor"
    n37 = node-c288() -> (→"Hall data gathering duration(us)":i64)  [unwired: 1 in]
    n38 = call <extravilib>:"Read.vi"("channel"=w113) -> ("element"=w112:bool)  [unwired: 1 in, 1 out]
    n39 = xnode "Read/Write Control"("FPGA VI Reference In"=w119, "error in"=w120) -> ("FPGA VI Reference Out"=w117:refnum<k20>, "error out"=w116:errorcluster, "Hall Period"=→"Hall Period":u32, "Hall Detection"=→"Hall Detection":bool)
    n40 = node-c288() -> ()  [unwired: 1 in, 1 out]
  }
  n41 = node-c288() -> (w34:T12)  [unwired: 4 in]
  n42 = flat-sequence {
    tunnel: [w132] -> w42
    tunnel: w21 -> [w130]
    tunnel: w11 -> [w126]
    tunnel: [w125] -> w10
    tunnel: w2 -> [w124]
    tunnel: [w124] -> w3
    tunnel: w42 -> [w218]
    tunnel: [w215] -> w12
    tunnel: w11 -> [w212]
    tunnel: w10 -> [w211]
    tunnel: [w210] -> w9
    tunnel: [w209] -> w6
    tunnel: w3 -> [w208]
    tunnel: [w292] -> w17
    tunnel: w9 -> [w287]
    tunnel: [w286] -> w7
    tunnel: w6 -> [w285]
    frame #0 {
      # "Set forward RPM to 0"
      # "Init the Motors"
      n43 = while {
        tunnel: w126 -> [w134]
        stop <- w137 stop-if-true
        n44 = call <extravilib>:"Read.vi"("channel"=w134) -> ("element"=w135:bool)  [unwired: 1 in, 1 out]
        n45 = Or(x="GO", y=w135) -> (x .or. y?=w137:bool)
      }
      n46 = xnode "PWM 2"("Duty Cycle"=0.5, "Frequency [Hz]"=4000, "error in (no error)"=w130) -> ("error out"=w133:errorcluster)
      n47 = xnode "Digital output (1 sample) 2"("B/DIO4 (Pin 19)"=FALSE ("B/DIO1 (Pin 13)"), "error in (no error)"=w133) -> ("error out"=w132:errorcluster)
      n48 = call "VescSetRpm.vi"("Speed (rpm)"=0) -> ("error out"=w125:errorcluster)  [unwired: 10 in]
    }
    frame #1 {
      # "Controlling the Motors"
      n49 = xnode "Digital output (1 sample) 3"("B/DIO4 (Pin 19)"=TRUE ("B/DIO1 (Pin 13)"), "error in (no error)"=w218) -> ("error out"=w214:errorcluster)
      n50 = node-c288() -> (w217:T12)  [unwired: 4 in]
      n51 = timed-loop {
        tunnel: w214 -> [w234]
        timing: w217 -> [_]
        timing-out: [_] -> w216
        tunnel: w212 -> [w236]
        tunnel: [w233] -> w209
        tunnel: w208 -> [w232]
        stop <- w243 stop-if-true
        # "Control Steering motor\nbased on IMU and PID values"
        # "Steering Motor"
        n52 = node-c288() -> (→"Steering Motor duration(us)":i64)  [unwired: 1 in]
        n53 = local read "Encoder Position (Counts)"() -> (w240:i32)
        n54 = call <extravilib>:"Read.vi"("channel"=w236) -> ("element"=w243:bool)  [unwired: 1 in, 1 out]
        n55 = local read "IMU Gyro Chart"() -> (w241:cluster{dbl, dbl, dbl})
        n56 = Get Date/Time In Seconds() -> (seconds since 1Jan1904=w227:timestamp)
        n57 = call "SteeringControl.vi"("Position (Counts)"=w240, "Cluster"=w241, "Limit"="Angle limit", "P gain"="P", "I gain"="I", "error in (no error)"=w234, "D gain"="D") -> ("error out"=w233:errorcluster, "PWM Out"=w229:dbl)  [unwired: 19 in]
        "Duty Cycle" <- w229
        n58 = To Double Precision Float(number=w227) -> (double precision float=w228:dbl)
        n59 = Build Array(w228, w229) -> (w230:dbl[])
        n60 = TDMS Write(0:w232, 1:enum16{"decimated", "interleaved"}."interleaved" ("data layout (0:decimated)"), 5:"Steering motor" ("group name in (Untitled)"), 7:string[] ["Time", "PWM"] ("channel name(s) in (Untitled)"), 9:w230) -> ()  [unwired: 1 in, 4 out]
        n61 = node-c288() -> ()  [unwired: 1 in, 1 out]
      }
      n62 = node-c288(w216) -> (w215:i64)
      n63 = while "Timed Loop" {
        tunnel: w212 -> [w222]
        tunnel: w211 -> [w220]
        tunnel: [w219] -> w210
        stop <- w223 stop-if-true
        # "Control forward\nmotor based on RPM"
        # "Forward Motor"
        n64 = call "VescSetRpm.vi"("error in (no error)"=w220, "Speed (rpm)"="Speed (rpm)") -> ("error out"=w219:errorcluster)  [unwired: 9 in]
        n65 = Wait (ms)(milliseconds to wait=1000) -> ()  [unwired: 1 out]
        n66 = call <extravilib>:"Read.vi"("channel"=w222) -> ("element"=w223:bool)  [unwired: 1 in, 1 out]
      }
    }
    frame #2 {
      # "Set forward RPM to 0"
      # "Turns off the motors"
      n67 = xnode "PWM 3"("Duty Cycle"=0.5, "Frequency [Hz]"=4000, "error in (no error)"=w285) -> ("error out"=w289:errorcluster)
      n68 = call "VescSetRpm.vi"("error in (no error)"=w287, "Speed (rpm)"=0) -> ("error out"=w286:errorcluster)  [unwired: 9 in]
      n69 = xnode "Digital output (1 sample)"("B/DIO4 (Pin 19)"=FALSE ("B/DIO1 (Pin 13)"), "error in (no error)"=w289) -> ("error out"=w292:errorcluster)
    }
  }
  n70 = timed-loop {
    tunnel: [w374] -> w19
    tunnel: w24 -> [w373]
    tunnel: w23 -> [w372]
    tunnel: [w370] -> w22
    timing: w34 -> [_]
    timing-out: [_] -> w33
    tunnel: w11 -> [w368]
    stop <- w371 stop-if-true
    # "GPS Receive data"
    n71 = node-c288() -> (→"GPS loop duration (us)":i64)  [unwired: 1 in]
    n72 = control-ref of="Raw output from GPS"() -> (w366:refnum<vi>)
    n73 = call <extravilib>:"Read.vi"("channel"=w368) -> ("element"=w367:bool)  [unwired: 1 in, 1 out]
    n74 = call "GPS.vi"("error in (no error)"=w372, "reference"=w366, "VISA Refnum"=w373) -> ("error out"=w370:errorcluster, "Array"=w375:string[], "Raw output from GPS"=→"Raw output from GPS":string, "VISA Refnum"=w374:refnum<visa-resource-name>, "read buffer"=w364:string)  [unwired: 4 in]
    n75 = Or(x=w370, y=w367) -> (x .or. y?=w371:bool)
    n76 = case shown="\"$GNRMC\"" w364 {
      tunnel: w375 -> [_ w393 w394 w444 w494 w554 w566 w583 w604 w605]
      frame "False", Default {
      }
      frame "$GNRMC" {
        n77 = Index Array(array=w393) -> (element #1=→"xxRMC":string, element #2=→"UTC Time":string, element #3=→"Status":string, element #4=→"Lat":string, element #5=→"N/S":string, element #6=→"Long":string, element #7=→"E/W":string, element #8=→"Speed over ground[knot]":string, element #9=→"Course over Ground [Degrees]":string, element #10=→"date[ddmmyy]":string, element #11=→"Mode":string, element #12=→"NavStatus":string, element #13=→"Checksum":string, element #14=→"Carriage return":string)  [unwired: 14 in]
      }
      frame "$GLGSV" {
        n78 = Index Array(array=w394) -> (element #1=→"GLGSV 2":string, element #2=→"number of message 2":string, element #3=w396:string, element #4=→"Satelite in view 2":string)  [unwired: 4 in]
        "msg1 2" <- w396
        n79 = Decimal String To Number(string=w396) -> (number=w395:i32)  [unwired: 2 in, 1 out]
        n80 = case shown="1" w395 {
          tunnel: w394 -> [_ w401 w411 w422 w433]
          frame 0, Default {
          }
          frame 1 {
            n81 = Array Subset(array=w401, index=4) -> (w406:string[])  [unwired: 1 in]
            "Satelite_id/elevation/azimuth/SNR 21" <- w406
            n82 = Array Subset(array=w406, index=4) -> (w407:string[])  [unwired: 1 in]
            "Satelite_id/elevation/azimuth/SNR 20" <- w407
            n83 = Array Subset(array=w407, index=4) -> (w408:string[])  [unwired: 1 in]
            "Satelite_id/elevation/azimuth/SNR 19" <- w408
            n84 = Array Subset(array=w408, index=4) -> (w410:string[])  [unwired: 1 in]
            "Satelite_id/elevation/azimuth/SNR 18" <- w410
            n85 = Array Subset(array=w410, index=4) -> (→"Signal ID / Check sum 5":string[])  [unwired: 1 in]
          }
          frame 2 {
            n86 = Array Subset(array=w411, index=4) -> (w417:string[])  [unwired: 1 in]
            "Satelite_id/elevation/azimuth/SNR 24" <- w417
            n87 = Array Subset(array=w417, index=4) -> (w418:string[])  [unwired: 1 in]
            "Satelite_id/elevation/azimuth/SNR 23" <- w418
            n88 = Array Subset(array=w418, index=4) -> (w419:string[])  [unwired: 1 in]
            "Satelite_id/elevation/azimuth/SNR 22" <- w419
            n89 = Array Subset(array=w419, index=4) -> (w421:string[])  [unwired: 1 in]
            "Satelite_id/elevation/azimuth/SNR 25" <- w421
            n90 = Array Subset(array=w421, index=4) -> (→"Signal ID / Check sum 6":string[])  [unwired: 1 in]
          }
          frame 3 {
            n91 = Array Subset(array=w422, index=4) -> (w428:string[])  [unwired: 1 in]
            "Satelite_id/elevation/azimuth/SNR 28" <- w428
            n92 = Array Subset(array=w428, index=4) -> (w429:string[])  [unwired: 1 in]
            "Satelite_id/elevation/azimuth/SNR 27" <- w429
            n93 = Array Subset(array=w429, index=4) -> (w430:string[])  [unwired: 1 in]
            "Satelite_id/elevation/azimuth/SNR 26" <- w430
            n94 = Array Subset(array=w430, index=4) -> (w432:string[])  [unwired: 1 in]
            "Satelite_id/elevation/azimuth/SNR 29" <- w432
            n95 = Array Subset(array=w432, index=4) -> (→"Signal ID / Check sum 7":string[])  [unwired: 1 in]
          }
          frame 4 {
            n96 = Array Subset(array=w433, index=4) -> (w439:string[])  [unwired: 1 in]
            "Satelite_id/elevation/azimuth/SNR 32" <- w439
            n97 = Array Subset(array=w439, index=4) -> (w440:string[])  [unwired: 1 in]
            "Satelite_id/elevation/azimuth/SNR 31" <- w440
            n98 = Array Subset(array=w440, index=4) -> (w441:string[])  [unwired: 1 in]
            "Satelite_id/elevation/azimuth/SNR 30" <- w441
            n99 = Array Subset(array=w441, index=4) -> (w443:string[])  [unwired: 1 in]
            "Satelite_id/elevation/azimuth/SNR 33" <- w443
            n100 = Array Subset(array=w443, index=4) -> (→"Signal ID / Check sum 8":string[])  [unwired: 1 in]
          }
        }
      }
      frame "$GAGSV" {
        n101 = Index Array(array=w444) -> (element #1=→"GAGSV 3":string, element #2=→"number of message 3":string, element #3=w446:string, element #4=→"Satelite in view 3":string)  [unwired: 4 in]
        "msg1 3" <- w446
        n102 = Decimal String To Number(string=w446) -> (number=w445:i32)  [unwired: 2 in, 1 out]
        n103 = case shown="1" w445 {
          tunnel: w444 -> [_ w451 w461 w472 w483]
          frame 0, Default {
          }
          frame 1 {
            n104 = Array Subset(array=w451, index=4) -> (w456:string[])  [unwired: 1 in]
            "Satelite_id/elevation/azimuth/SNR 38" <- w456
            n105 = Array Subset(array=w456, index=4) -> (w457:string[])  [unwired: 1 in]
            "Satelite_id/elevation/azimuth/SNR 37" <- w457
            n106 = Array Subset(array=w457, index=4) -> (w458:string[])  [unwired: 1 in]
            "Satelite_id/elevation/azimuth/SNR 36" <- w458
            n107 = Array Subset(array=w458, index=4) -> (w460:string[])  [unwired: 1 in]
            "Satelite_id/elevation/azimuth/SNR 35" <- w460
            n108 = Array Subset(array=w460, index=4) -> (→"Signal ID / Check sum 9":string[])  [unwired: 1 in]
          }
          frame 2 {
            n109 = Array Subset(array=w461, index=4) -> (w467:string[])  [unwired: 1 in]
            "Satelite_id/elevation/azimuth/SNR 41" <- w467
            n110 = Array Subset(array=w467, index=4) -> (w468:string[])  [unwired: 1 in]
            "Satelite_id/elevation/azimuth/SNR 40" <- w468
            n111 = Array Subset(array=w468, index=4) -> (w469:string[])  [unwired: 1 in]
            "Satelite_id/elevation/azimuth/SNR 39" <- w469
            n112 = Array Subset(array=w469, index=4) -> (w471:string[])  [unwired: 1 in]
            "Satelite_id/elevation/azimuth/SNR 42" <- w471
            n113 = Array Subset(array=w471, index=4) -> (→"Signal ID / Check sum 10":string[])  [unwired: 1 in]
          }
          frame 3 {
            n114 = Array Subset(array=w472, index=4) -> (w478:string[])  [unwired: 1 in]
            "Satelite_id/elevation/azimuth/SNR 45" <- w478
            n115 = Array Subset(array=w478, index=4) -> (w479:string[])  [unwired: 1 in]
            "Satelite_id/elevation/azimuth/SNR 44" <- w479
            n116 = Array Subset(array=w479, index=4) -> (w480:string[])  [unwired: 1 in]
            "Satelite_id/elevation/azimuth/SNR 43" <- w480
            n117 = Array Subset(array=w480, index=4) -> (w482:string[])  [unwired: 1 in]
            "Satelite_id/elevation/azimuth/SNR 46" <- w482
            n118 = Array Subset(array=w482, index=4) -> (→"Signal ID / Check sum 11":string[])  [unwired: 1 in]
          }
          frame 4 {
            n119 = Array Subset(array=w483, index=4) -> (w489:string[])  [unwired: 1 in]
            "Satelite_id/elevation/azimuth/SNR 49" <- w489
            n120 = Array Subset(array=w489, index=4) -> (w490:string[])  [unwired: 1 in]
            "Satelite_id/elevation/azimuth/SNR 48" <- w490
            n121 = Array Subset(array=w490, index=4) -> (w491:string[])  [unwired: 1 in]
            "Satelite_id/elevation/azimuth/SNR 47" <- w491
            n122 = Array Subset(array=w491, index=4) -> (w493:string[])  [unwired: 1 in]
            "Satelite_id/elevation/azimuth/SNR 50" <- w493
            n123 = Array Subset(array=w493, index=4) -> (→"Signal ID / Check sum 12":string[])  [unwired: 1 in]
          }
        }
      }
      frame "$GBGSV" {
        n124 = Index Array(array=w494) -> (element #1=→"GBGSV 4":string, element #2=→"number of message 4":string, element #3=w496:string, element #4=→"Satelite in view 4":string)  [unwired: 4 in]
        "msg1 4" <- w496
        n125 = Decimal String To Number(string=w496) -> (number=w495:i32)  [unwired: 2 in, 1 out]
        n126 = case shown="1" w495 {
          tunnel: w494 -> [_ w501 w511 w522 w533]
          frame 0, Default {
          }
          frame 1 {
            n127 = Array Subset(array=w501, index=4) -> (w506:string[])  [unwired: 1 in]
            "Satelite_id/elevation/azimuth/SNR 55" <- w506
            n128 = Array Subset(array=w506, index=4) -> (w507:string[])  [unwired: 1 in]
            "Satelite_id/elevation/azimuth/SNR 54" <- w507
            n129 = Array Subset(array=w507, index=4) -> (w508:string[])  [unwired: 1 in]
            "Satelite_id/elevation/azimuth/SNR 53" <- w508
            n130 = Array Subset(array=w508, index=4) -> (w510:string[])  [unwired: 1 in]
            "Satelite_id/elevation/azimuth/SNR 52" <- w510
            n131 = Array Subset(array=w510, index=4) -> (→"Signal ID / Check sum 13":string[])  [unwired: 1 in]
          }
          frame 2 {
            n132 = Array Subset(array=w511, index=4) -> (w517:string[])  [unwired: 1 in]
            "Satelite_id/elevation/azimuth/SNR 58" <- w517
            n133 = Array Subset(array=w517, index=4) -> (w518:string[])  [unwired: 1 in]
            "Satelite_id/elevation/azimuth/SNR 57" <- w518
            n134 = Array Subset(array=w518, index=4) -> (w519:string[])  [unwired: 1 in]
            "Satelite_id/elevation/azimuth/SNR 56" <- w519
            n135 = Array Subset(array=w519, index=4) -> (w521:string[])  [unwired: 1 in]
            "Satelite_id/elevation/azimuth/SNR 59" <- w521
            n136 = Array Subset(array=w521, index=4) -> (→"Signal ID / Check sum 14":string[])  [unwired: 1 in]
          }
          frame 3 {
            n137 = Array Subset(array=w522, index=4) -> (w528:string[])  [unwired: 1 in]
            "Satelite_id/elevation/azimuth/SNR 62" <- w528
            n138 = Array Subset(array=w528, index=4) -> (w529:string[])  [unwired: 1 in]
            "Satelite_id/elevation/azimuth/SNR 61" <- w529
            n139 = Array Subset(array=w529, index=4) -> (w530:string[])  [unwired: 1 in]
            "Satelite_id/elevation/azimuth/SNR 60" <- w530
            n140 = Array Subset(array=w530, index=4) -> (w532:string[])  [unwired: 1 in]
            "Satelite_id/elevation/azimuth/SNR 63" <- w532
            n141 = Array Subset(array=w532, index=4) -> (→"Signal ID / Check sum 15":string[])  [unwired: 1 in]
          }
          frame 4 {
            n142 = Array Subset(array=w533, index=4) -> (w539:string[])  [unwired: 1 in]
            "Satelite_id/elevation/azimuth/SNR 66" <- w539
            n143 = Array Subset(array=w539, index=4) -> (w540:string[])  [unwired: 1 in]
            "Satelite_id/elevation/azimuth/SNR 65" <- w540
            n144 = Array Subset(array=w540, index=4) -> (w541:string[])  [unwired: 1 in]
            "Satelite_id/elevation/azimuth/SNR 64" <- w541
            n145 = Array Subset(array=w541, index=4) -> (w543:string[])  [unwired: 1 in]
            "Satelite_id/elevation/azimuth/SNR 67" <- w543
            n146 = Array Subset(array=w543, index=4) -> (→"Signal ID / Check sum 16":string[])  [unwired: 1 in]
          }
        }
      }
      frame "$GNGLL" {
        n147 = Index Array(array=w554) -> (element #1=→"GLL":string, element #2=→"Lat 2":string, element #3=→"NS":string, element #4=→"Long 3":string, element #5=→"EW":string, element #6=→"Time":string, element #7=→"Status 2":string, element #8=→"Positioning mod":string, element #9=→"Check sum":string, element #10=→"Carriage return 2":string)  [unwired: 10 in]
      }
      frame "$GNVTG" {
        n148 = Index Array(array=w566) -> (element #1=→"VTG":string, element #2=→"Course over Ground":string, element #3=→"Reference":string, element #4=→"Course over Ground (Magnetic)":string, element #5=→"Reference2":string, element #6=→"Speedover Ground (knots)":string, element #7=→"Units1":string, element #8=→"Speed over ground kph":string, element #9=→"Units 2":string, element #10=→"Position Mode 2":string, element #11=→"Check sum 2":string)  [unwired: 11 in]
      }
      frame "$GNGGA" {
        n149 = Index Array(array=w583) -> (element #1=→"GGA 3":string, element #2=→"UTC time":string, element #3=→"Lat 3":string, element #4=→"NS 2":string, element #5=→"Long 2":string, element #6=→"EW 2":string, element #7=→"Pos_indicator":string, element #8=→"Number of Satelite_used":string, element #9=→"hdop":string, element #10=→"msl_altitude":string, element #11=→"altitude_units":string, element #12=→"geoidal_Seperation":string, element #13=→"Separation unit":string, element #14=→"age of Diff corr":string, element #15=→"diffStating":string, element #16=→"Checksum 2":string)  [unwired: 16 in]
      }
      frame "$GNGSA" {
        n150 = Index Array(array=w604) -> (element #1=→"GSA":string, element #2=→"Operation Mode":string, element #3=→"Navigation mode":string, element #4=→"satelite used channel 1":string, element #5=→"satelite used channel 2":string, element #6=→"satelite used channel 3":string, element #7=→"satelite used channel 4":string, element #8=→"satelite used channel 5":string, element #9=→"satelite used channel 6":string, element #10=→"satelite used channel 7":string, element #11=→"satelite used channel 8":string, element #12=→"satelite used channel 9":string, element #13=→"satelite used channel 10":string, element #14=→"satelite used channel 11":string, element #15=→"satelite used channel 12":string, element #16=→"pdop":string, element #17=→"hdop 2":string, element #18=→"vdop":string, element #19=→"System ID":string, element #20=→"Checksum 3":string)  [unwired: 20 in]
      }
      frame "$GPGSV" {
        n151 = Index Array(array=w605) -> (element #1=→"GPGSV":string, element #2=→"number of message":string, element #3=w607:string, element #4=→"Satelite in view":string)  [unwired: 4 in]
        "msg1" <- w607
        n152 = Decimal String To Number(string=w607) -> (number=w606:i32)  [unwired: 2 in, 1 out]
        n153 = case shown="1" w606 {
          tunnel: w605 -> [_ w612 w622 w633 w644]
          frame 0, Default {
          }
          frame 1 {
            n154 = Array Subset(array=w612, index=4) -> (w617:string[])  [unwired: 1 in]
            "Satelite_id/elevation/azimuth/SNR" <- w617
            n155 = Array Subset(array=w617, index=4) -> (w618:string[])  [unwired: 1 in]
            "Satelite_id/elevation/azimuth/SNR 2" <- w618
            n156 = Array Subset(array=w618, index=4) -> (w619:string[])  [unwired: 1 in]
            "Satelite_id/elevation/azimuth/SNR 3" <- w619
            n157 = Array Subset(array=w619, index=4) -> (w621:string[])  [unwired: 1 in]
            "Satelite_id/elevation/azimuth/SNR 4" <- w621
            n158 = Array Subset(array=w621, index=4) -> (→"Signal ID / Check sum":string[])  [unwired: 1 in]
          }
          frame 2 {
            n159 = Array Subset(array=w622, index=4) -> (w628:string[])  [unwired: 1 in]
            "Satelite_id/elevation/azimuth/SNR 5" <- w628
            n160 = Array Subset(array=w628, index=4) -> (w629:string[])  [unwired: 1 in]
            "Satelite_id/elevation/azimuth/SNR 6" <- w629
            n161 = Array Subset(array=w629, index=4) -> (w630:string[])  [unwired: 1 in]
            "Satelite_id/elevation/azimuth/SNR 7" <- w630
            n162 = Array Subset(array=w630, index=4) -> (w632:string[])  [unwired: 1 in]
            "Satelite_id/elevation/azimuth/SNR 8" <- w632
            n163 = Array Subset(array=w632, index=4) -> (→"Signal ID / Check sum 2":string[])  [unwired: 1 in]
          }
          frame 3 {
            n164 = Array Subset(array=w633, index=4) -> (w639:string[])  [unwired: 1 in]
            "Satelite_id/elevation/azimuth/SNR 9" <- w639
            n165 = Array Subset(array=w639, index=4) -> (w640:string[])  [unwired: 1 in]
            "Satelite_id/elevation/azimuth/SNR 10" <- w640
            n166 = Array Subset(array=w640, index=4) -> (w641:string[])  [unwired: 1 in]
            "Satelite_id/elevation/azimuth/SNR 11" <- w641
            n167 = Array Subset(array=w641, index=4) -> (w643:string[])  [unwired: 1 in]
            "Satelite_id/elevation/azimuth/SNR 12" <- w643
            n168 = Array Subset(array=w643, index=4) -> (→"Signal ID / Check sum 3":string[])  [unwired: 1 in]
          }
          frame 4 {
            n169 = Array Subset(array=w644, index=4) -> (w650:string[])  [unwired: 1 in]
            "Satelite_id/elevation/azimuth/SNR 13" <- w650
            n170 = Array Subset(array=w650, index=4) -> (w651:string[])  [unwired: 1 in]
            "Satelite_id/elevation/azimuth/SNR 14" <- w651
            n171 = Array Subset(array=w651, index=4) -> (w652:string[])  [unwired: 1 in]
            "Satelite_id/elevation/azimuth/SNR 15" <- w652
            n172 = Array Subset(array=w652, index=4) -> (w654:string[])  [unwired: 1 in]
            "Satelite_id/elevation/azimuth/SNR 16" <- w654
            n173 = Array Subset(array=w654, index=4) -> (→"Signal ID / Check sum 4":string[])  [unwired: 1 in]
          }
        }
      }
    }
    n174 = node-c288() -> ()  [unwired: 1 in, 1 out]
  }
  n175 = node-c288(w43) -> (w41:i64)
  n176 = node-c288(w52) -> (w40:i64)
  n177 = node-c288(w45) -> (w14:i64)
  n178 = call <vilib>:"Close.vi"("error in (no error)"=w16, "I2C Ref In"=w20) -> ("error out"=w18:errorcluster)  [unwired: 9 in]
  n179 = node-c288(w50) -> (w39:i64)
  n180 = node-c288(w33) -> (w13:i64)
  n181 = VISA Flush I/O Buffer(VISA resource name=w19, error in (no error)=w22) -> (VISA resource name out=w26:refnum<visa-resource-name>, error out=w25:errorcluster)  [unwired: 1 in]
  n182 = VISA Close(VISA resource name=w26, error in (no error)=w25) -> (error out=w8:errorcluster)
  n183 = Merge Errors(w49, w48, w18, w17, w7, w8) -> (w47:errorcluster)
  n184 = call <vilib>:"Simple Error Handler.vi"("error in (no error)"=w47) -> ("error out"=w1:errorcluster)  [unwired: 4 in, 4 out]
  n185 = TDMS Close(8:w1, 11:w2) -> ()  [unwired: 2 out]
  n186 = xnode "Invoke Method"("FPGA VI Reference In"=w54, "error in"=w1) -> ("FPGA VI Reference Out"=w57:refnum<k20>, "error out"=w55:errorcluster)
  n187 = call <vilib>:"Reset myRIO.vi"("error in (no error)"=w55) -> ("error out"=w56:errorcluster)  [unwired: 10 in]
  n188 = xnode "Close FPGA VI Reference"("FPGA VI Reference In"=w57, "error in"=w56) -> ()  [unwired: 1 out]
  n189 = Compound Arithmetic op=ADD(w41, w40, w39, w14, w13, w12) -> (→"Combined loop duration time (us)":i64)
